vi "Addon.Version.Upgrade.vi"(8 "error in (no error)":errorcluster, 11 "Device Item Ref in in":T1 format="%.0x") -> (0 "error out":errorcluster, 3 "Device Item Ref out":T1 format="%.0x")   [LabVIEW 2019, in "Diagnostics Addon Shared.lvlib"]
uses:
  Diagnostics Addon Shared.lvlib
  <vilib>/NI VeriStand/Custom Device API/Custom Device Item Ref.ctl
  Types/Security.Type.ctl
  Types/Settings.Channel.ctl
  <vilib>/NI VeriStand/Custom Device API/Custom Device Channel.ctl
  <vilib>/NI VeriStand/Custom Device API/Custom Device Channel Type.ctl
  NationalInstruments.VeriStand.SystemDefinitionAPI
  Constants.vi
  <vilib>/NI/NI VeriStand Advanced SysDef API/_SubVIs/SysDef.Search.GUID.vi
  <vilib>/NI/NI VeriStand Advanced SysDef API/_SubVIs/SysDef.Property.Get.U32.vi
  <vilib>/NI/NI VeriStand Advanced SysDef API/_SubVIs/SysDef.Property.Get.String.vi
  <vilib>/NI VeriStand/Custom Device API/Custom Device API.lvlib
  <vilib>/NI/NI VeriStand Advanced SysDef API/SysDef API/Advanced System Definition.lvlib
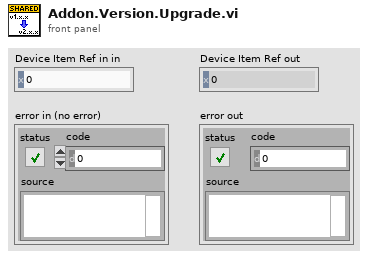
[diagram p1: front panel]
types:
  T1 = typedef "Custom Device API.lvlib/Custom Device Item Ref.ctl" = u64
  T2 = typedef "Diagnostics Addon Shared.lvlib/Security.Type.ctl" = enum16{"None", "DLL", "MasterKey"}
  T3 = typedef "Diagnostics Addon Shared.lvlib/Settings.Channel.ctl" = cluster{"Name":string, "Description":string, "Channel":T4}
  T4 = typedef "Custom Device API.lvlib/Custom Device Channel.ctl" = cluster{"Type":T5, "Units":string, "Default Value":dbl, "Faultable":bool, "Scalable":bool}
  T5 = typedef "Custom Device API.lvlib/Custom Device Channel Type.ctl" = enum16{"Input", "Output"}
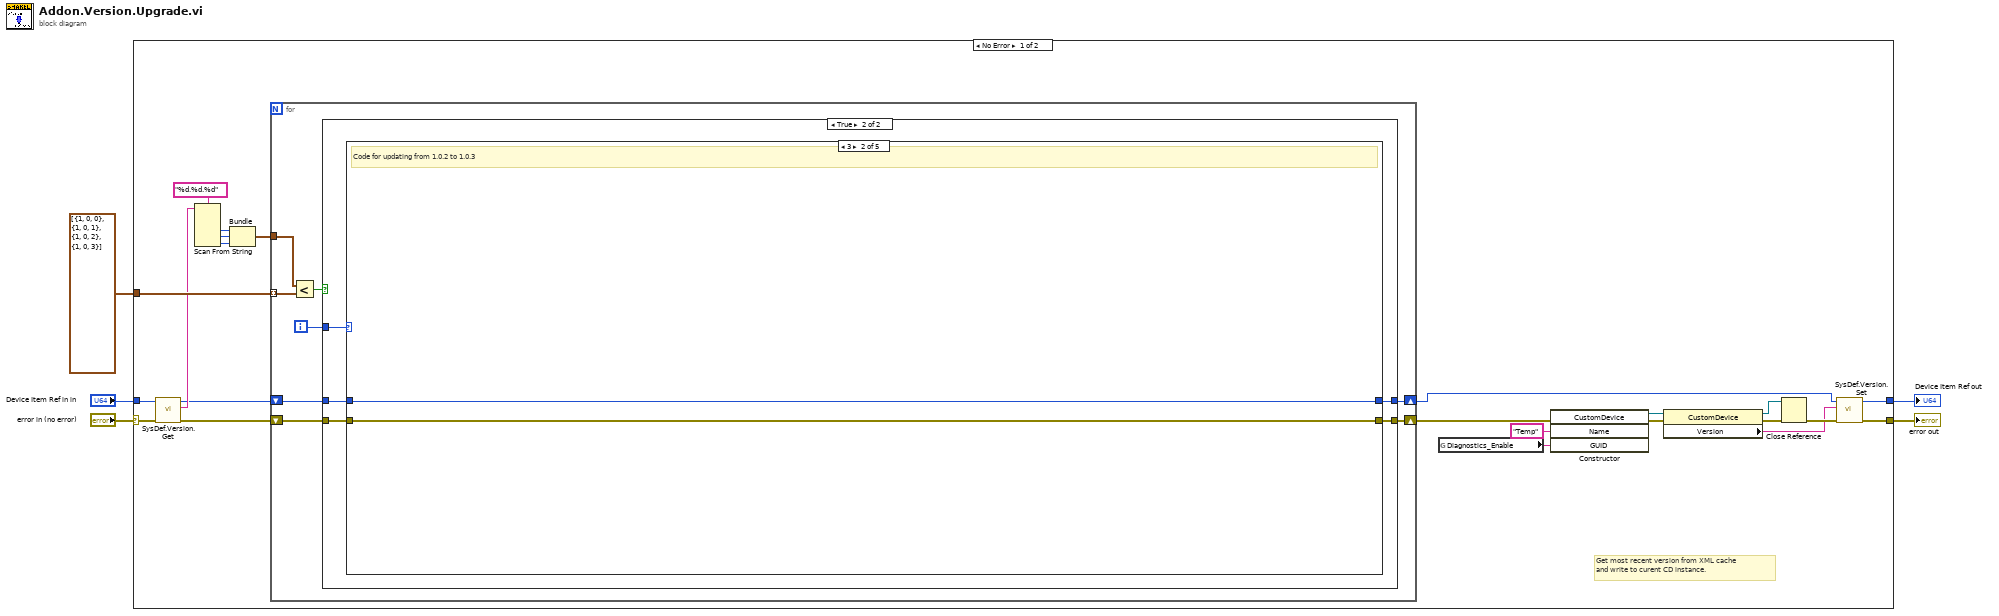
[diagram p0: block diagram]
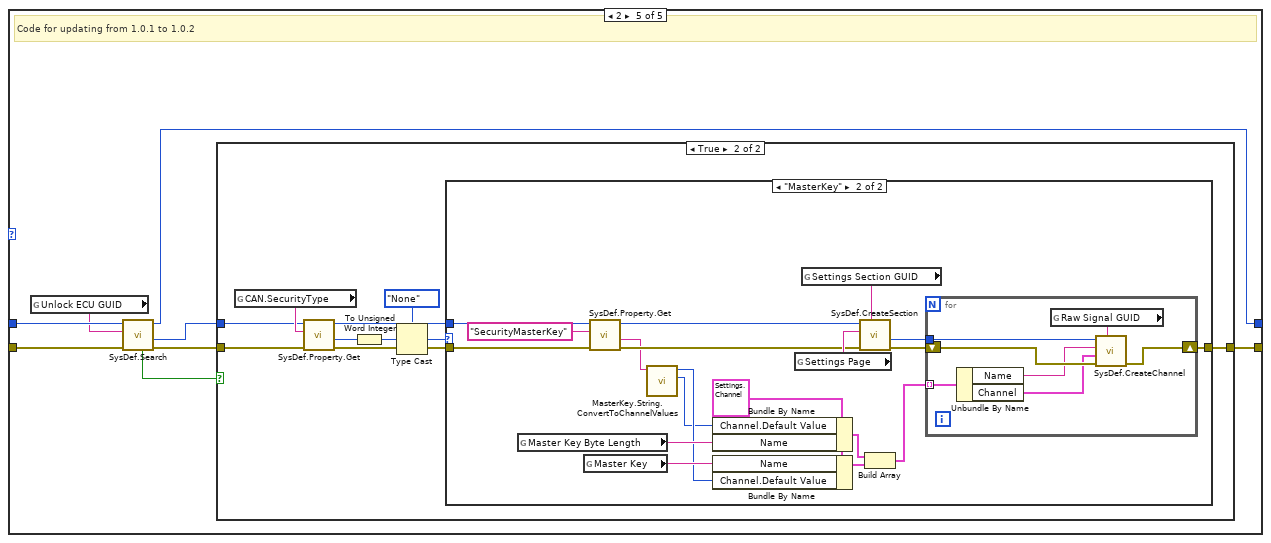
[diagram p6: hidden frame]
diagram:
  n1 = case shown="No Error" "error in (no error)" {
    selector: "error in (no error)" -> [w11 w99]
    tunnel: [w21 w99] -> w4
    tunnel: "Device Item Ref in in" -> [w10 w98]
    tunnel: [w20 w98] -> w5
    tunnel: cluster{i32, i32, i32}[] [{1, 0, 0}, {1, 0, 1}, {1, 0, 2}, {1, 0, 3}] -> [w28 _]
    frame No Error {
      # "Get most recent version from XML cache\nand write to curent CD instance."
      n2 = call <vilib>:"SysDef.Version.Get.vi"("error in (no error)"=w11, "nodeID"=w10) -> ("error out"=w7:errorcluster, "Version"=w15:string, "nodeID out"=w6:u64)  [unwired: 7 in]
      n3 = Scan From String(format string="%d.%d.%d", input string=w15) -> (output 1=w13:i32, output 2=w12:i32, output 3=w14:i32)  [unwired: 5 in, 3 out]
      n4 = Bundle(w13, w12, w14) -> (w8:cluster{i32, i32, i32})  [unwired: 1 in]
      n5 = for {
        tunnel: w28 -> [w34] mode=indexing
        shift-right: [w36] -> w19
        shift-left: w7 -> [w30]
        shift-right: [w35] -> w18
        shift-left: w6 -> [w29]
        tunnel: w8 -> [w31]
        i -> [w32]
        n6 = Less?(x=w31, y=w34) -> (x < y?=w33:bool)
        n7 = case shown="True" w33 {
          tunnel: w30 -> [w38 w43]
          tunnel: [w38 w42] -> w36
          tunnel: w29 -> [w37 w39]
          tunnel: [w37 w40] -> w35
          tunnel: w32 -> [_ w41]
          frame False {
          }
          frame True {
            n8 = case shown="3" w41 {
              tunnel: w43 -> [w45 w47 w49 w51 w59]
              tunnel: [w45 w47 w49 w51 w53] -> w42
              tunnel: [w44 w46 w48 w50 w58] -> w40
              tunnel: w39 -> [w44 w46 w48 w50 w57]
              frame Default {
                # "Nothing to update"
              }
              frame 3 {
                # "Code for updating from 1.0.2 to 1.0.3"
              }
              frame 0 {
                # "Initial Onload"
              }
              frame 1 {
                # "Code for updating from 1.0.0 to 1.0.1"
              }
              frame 2 {
                # "Code for updating from 1.0.1 to 1.0.2"
                n9 = global read "Constants.vi" "Unlock ECU GUID"() -> (w52:string)
                n10 = call-poly <vilib>:"SysDef.Search.vi"("error in (no error)"=w59, "GUID"=w52, "nodeID"=w57) -> ("error out"=w55:errorcluster, "Value out"=w54:u64, "nodeID out"=w58:u64, "Found?"=w56:bool)  [unwired: 5 in]
                n11 = case shown="True" w56 {
                  tunnel: w55 -> [w60 w65]
                  tunnel: w54 -> [_ w68]
                  tunnel: [w60 w70] -> w53
                  frame False {
                  }
                  frame True {
                    n12 = global read "Constants.vi" "CAN.SecurityType"() -> (w69:string)
                    n13 = call-poly <vilib>:"SysDef.Property.Get.vi"("error in (no error)"=w65, "Property Name"=w69, "nodeID"=w68) -> ("error out"=w66:errorcluster, "Value out"=w64:u32, "nodeID out"=w67:u64)  [unwired: 5 in, 1 out]
                    n14 = To Unsigned Word Integer(number=w64) -> (unsigned 16bit integer=w63:u16)
                    n15 = Type Cast(type=Security.Type."None" ("Type"), x=w63) -> (*(type *) &x=w61:T2)
                    n16 = case shown="\"MasterKey\"" w61 {
                      tunnel: w66 -> [w71 w84]
                      tunnel: w67 -> [_ w83]
                      tunnel: [w71 w76] -> w70
                      frame Default {
                      }
                      frame "MasterKey" {
                        w86 = T3 {"Name"="Byte Length", "Description"="", "Channel"={"Type"=enum."Input", "Units"="", "Default Value"=0.0, "Faultable"=FALSE, "Scalable"=FALSE}} ("cluster")
                        n17 = global read "Constants.vi" "Master Key Byte Length"() -> (w88:string)
                        n18 = global read "Constants.vi" "Master Key"() -> (w87:string)
                        n19 = call-poly <vilib>:"SysDef.Property.Get.vi"("error in (no error)"=w84, "Property Name"="SecurityMasterKey" ("CAN.SecurityMasterKey"), "nodeID"=w83) -> ("error out"=w78:errorcluster, "Value out"=w75:string, "nodeID out"=w77:u64)  [unwired: 5 in, 1 out]
                        n20 = call "MasterKey.String.ConvertToChannelValues.vi"("Master Key"=w75) -> ("Length"=w72:i32, "Value"=w73:u64)  [unwired: 9 in]
                        n21 = Bundle By Name(cluster=w86, "Channel.Default Value"=w72, "Name"=w88) -> (w89:T3)
                        n22 = Bundle By Name(cluster=w86, "Name"=w87, "Channel.Default Value"=w73) -> (w90:T3)
                        n23 = global read "Constants.vi" "Settings Page"() -> (w82:string)
                        n24 = global read "Constants.vi" "Settings Section GUID"() -> (w81:string)
                        n25 = call <vilib>:"SysDef.CreateSection.vi"("GUID"=w81, "error in (no error)"=w78, "Name"=w82, "nodeID"=w77) -> ("error out"=w79:errorcluster, "New NodeID"=w80:u64)  [unwired: 4 in, 2 out]
                        n26 = Build Array(w89, w90) -> (w74:T3[])
                        n27 = for {
                          tunnel: w80 -> [w95]
                          shift-right: [w94] -> w76
                          shift-left: w79 -> [w96]
                          tunnel: w74 -> [w91] mode=indexing
                          n28 = Unbundle By Name(w91) -> ("Name"=w93:string, "Channel"=w92:T4)
                          n29 = global read "Constants.vi" "Raw Signal GUID"() -> (w97:string)
                          n30 = call <vilib>:"SysDef.CreateChannel.vi"("GUID"=w97, "error in (no error)"=w96, "Channel"=w92, "Name"=w93, "nodeID"=w95) -> ("error out"=w94:errorcluster)  [unwired: 3 in, 3 out]
                        }
                      }
                    }
                  }
                }
              }
            }
          }
        }
      }
      n31 = global read "Constants.vi" "Diagnostics_Enable"() -> (w16:string)
      n32 = constructor class="CustomDevice"(error in=w19, "Name"="Temp", "GUID"=w16) -> (reference out=w27:refnum<k24>, error out=w26:errorcluster)  [unwired: 2 in, 3 out]
      n33 = property class="CustomDevice"(reference=w27, error in=w26) -> (reference out=w24:refnum<k24>, error out=w25:errorcluster, "Version"=w22:string)
      n34 = Close Reference(reference=w24, error in (no error)=w25) -> (error out=w23:errorcluster)
      n35 = call <vilib>:"SysDef.Version.Set.vi"("error in (no error)"=w23, "Version"=w22, "nodeID"=w18) -> ("error out"=w21:errorcluster, "nodeID out"=w20:u64)  [unwired: 7 in]
    }
    frame Error {
    }
  }
  "Device Item Ref out" <- w5
  "error out" <- w4
